vi "Close.vi"(8 "error in (no error)":errorcluster, 11 "Devantech SRF05 in":refnum<class "Devantech SRF05.lvclass">) -> (0 "error out":errorcluster)   [LabVIEW 2019, in "Devantech SRF05.lvclass"]
doc: "Tterminating software connection."
uses:
  Devantech SRF05.lvclass
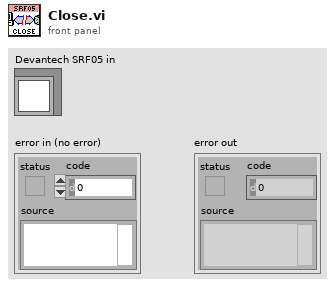
[diagram p1: front panel]
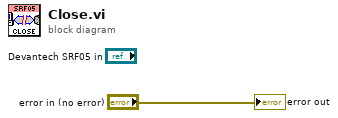
[diagram p0: block diagram]
diagram:
  "error out" <- "error in (no error)"
